vi "Test.vi"   [LabVIEW 2019]
doc: "This VI is called when test mode begins, and will automatically be terminated when it ends. You can add manual or automatic tests and invoke them from the dashboard."
uses:
  <vilib>/Rock Robotics/WPI/ThirdParty/Phoenix-LabVIEW/Motor Controller/Get/CTRE_Phoenix_MotorController_GetQuadratureData.vi
  <vilib>/Rock Robotics/WPI/Solenoid/Deprecated/WPI_SolenoidGetBool.vi
  <vilib>/Rock Robotics/WPI/Solenoid/WPI_SolenoidGetEnum.vi
types:
  T1 = typedef "WPI_SolenoidDevRef.ctl" = cluster{"DevStatus":errorcluster, "Pneumatics Control Module":u8, "Forward Solenoid Channel":T2, "Reverse Solenoid Channel":T2}
  T2 = typedef "WPI_SolenoidChannel.ctl" = enum8{"Solenoid 0", "Solenoid 1", "Solenoid 2", "Solenoid 3", "Solenoid 4", "Solenoid 5", "Solenoid 6", "Solenoid 7", "Invalid"}
  T3 = typedef "WPI_MotorControlDeviceRef.ctl" = cluster{"DeviceStatus":errorcluster, "Type":T4, "PWM":cluster{"PWM Channel":T5, "DeadBand":T6}, "CAN":cluster{"Device Number":u8, "SetOutput VI Ref":variant, "GetOutput VI Ref":variant, "Enable VI Ref":variant, "Disable VI Ref":variant, "Data":variant}, "Invert":bool, "DIO PWM":cluster{"PWM \"Enable\" Channel":T5, "DIOChannel":T7, "PWM Rate":dbl}}
  T4 = typedef "WPI_MotorControlType.ctl" = enum16{"PWM", "CAN", "DIO PWM"}
  T5 = typedef "FPGA_DIOPWMChannel.ctl" = enum8{"PWM 0", "PWM 1", "PWM 2", "PWM 3", "PWM 4", "PWM 5", "PWM 6", "PWM 7", "PWM 8", "PWM 9", "PWM MXP 0", "PWM MXP 1", "PWM MXP 2", "PWM MXP 3", "PWM MXP 4", "PWM MXP 5", "PWM MXP 6", "PWM MXP 7", "PWM MXP 8", "PWM MXP 9", "Invalid"}
  T6 = typedef "WPI_PWMDeadband.ctl" = cluster{"Name":string, "maxPositivePwm":i32, "minPositivePwm":i32, "centerPwm":i32, "maxNegativePwm":i32, "minNegativePwm":i32, "angularRange":u16}
  T7 = typedef "FPGA_DIOChannel.ctl" = enum8{"DIO 0", "DIO 1", "DIO 2", "DIO 3", "DIO 4", "DIO 5", "DIO 6", "DIO 7", "DIO 8", "DIO 9", "DIO MXP 0", "DIO MXP 1", "DIO MXP 2", "DIO MXP 3", "DIO MXP 4", "DIO MXP 5", "DIO MXP 6", "DIO MXP 7", "DIO MXP 8", "DIO MXP 9", "DIO MXP 10", "DIO MXP 11", "DIO MXP 12", "DIO MXP 13", "DIO MXP 14", "DIO MXP 15", "SPI Port CS1", "SPI Port CS2", "SPI Port CS3", "SPI Port MISO", "SPI Port MOSI", "Invalid"}
  T8 = typedef "WPI_SwitchDevRef.ctl" = cluster{"DevStatus":errorcluster, "DIO Channel":T7, "CntIndex":T9, "Normally Closed":bool}
  T9 = typedef "FPGA_CounterCtrSystemIndex.ctl" = enum8{"Ctr 0", "Ctr 1", "Ctr 2", "Ctr 3", "Ctr 4", "Ctr 5", "Ctr 6", "Ctr 7", "Invalid"}
  T10 = typedef "WPI_SolenoidValue.ctl" = enum16{"Off", "On", "Forward", "Reverse"}
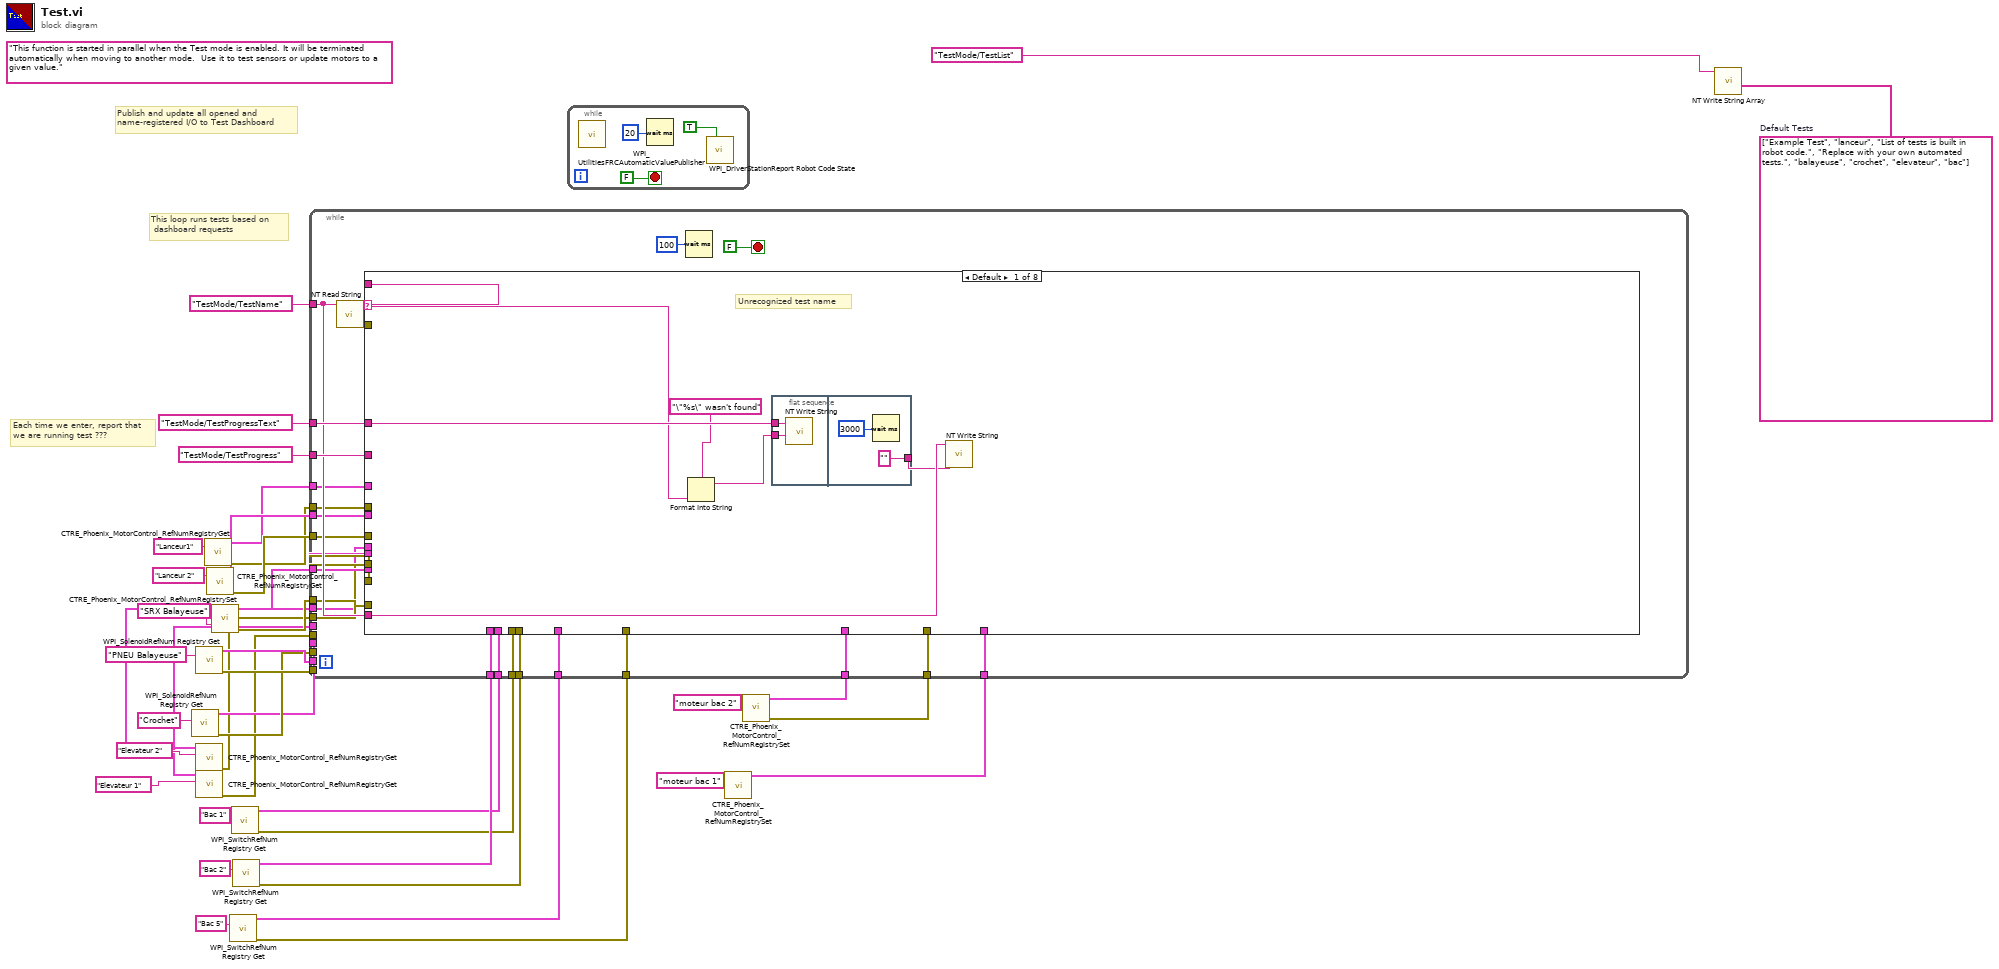
[diagram p0: block diagram]
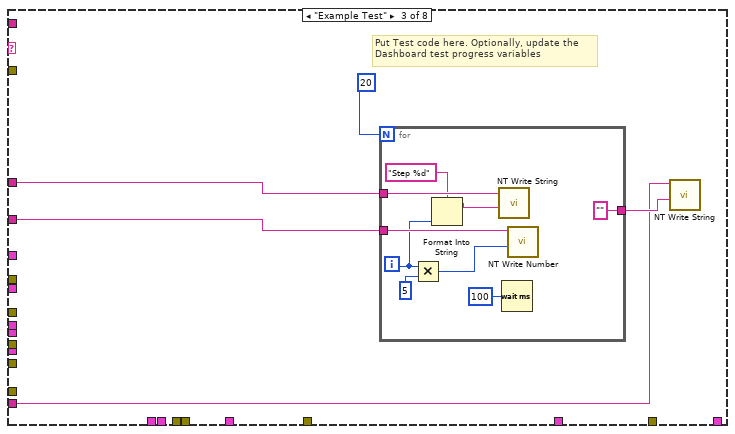
[diagram p3: hidden frame]
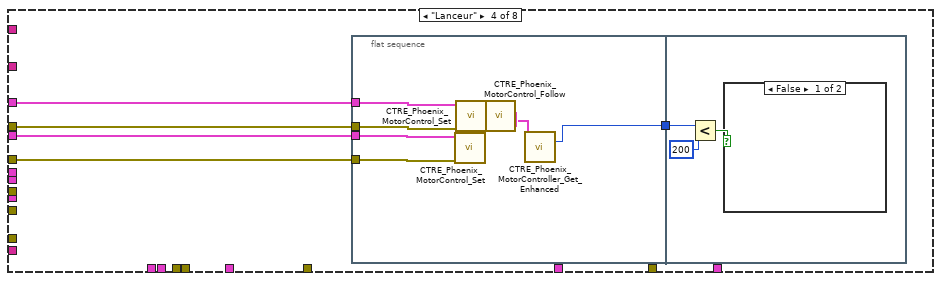
[diagram p4: hidden frame]
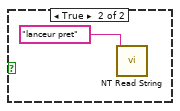
[diagram p5: hidden frame]
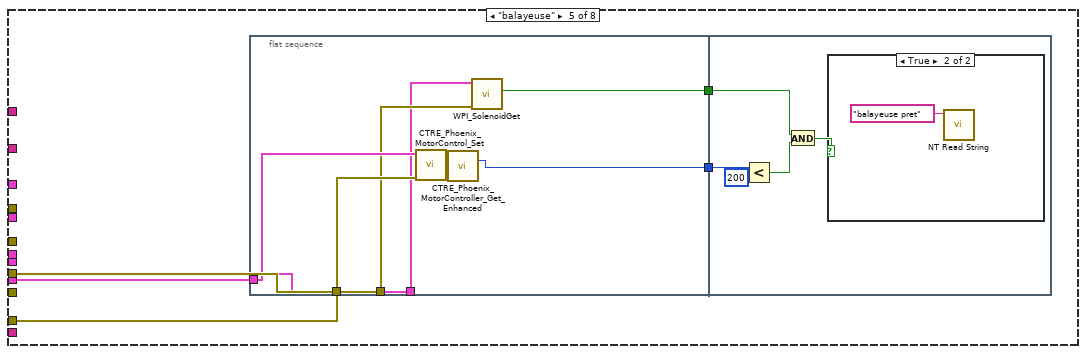
[diagram p6: hidden frame]
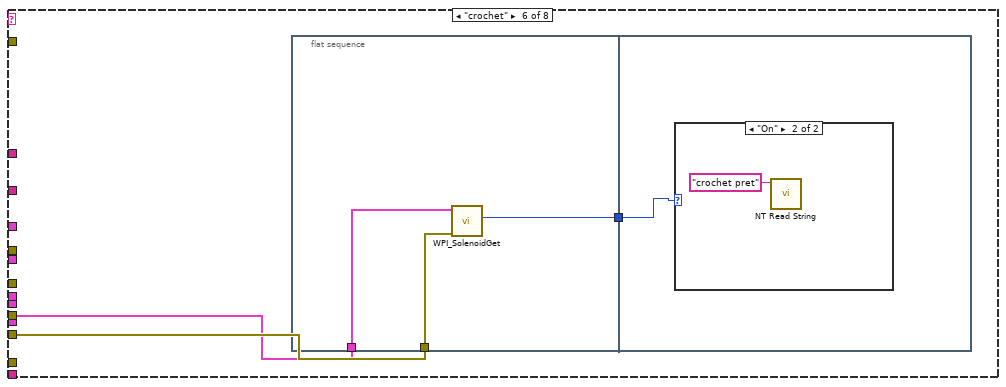
[diagram p8: hidden frame]
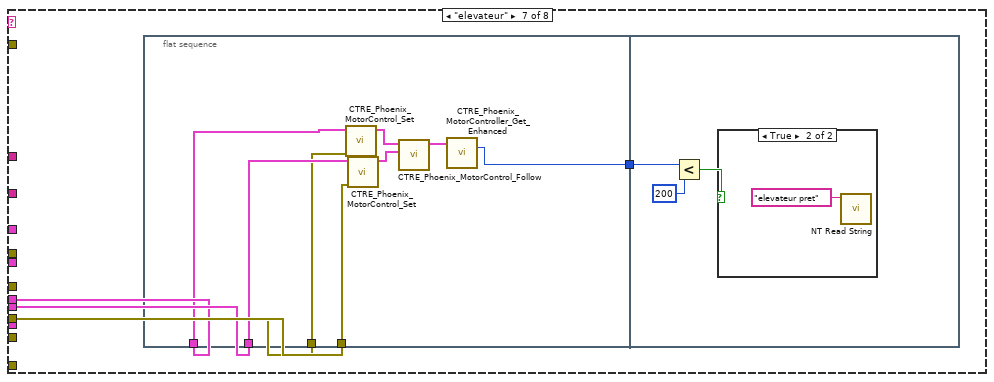
[diagram p10: hidden frame]
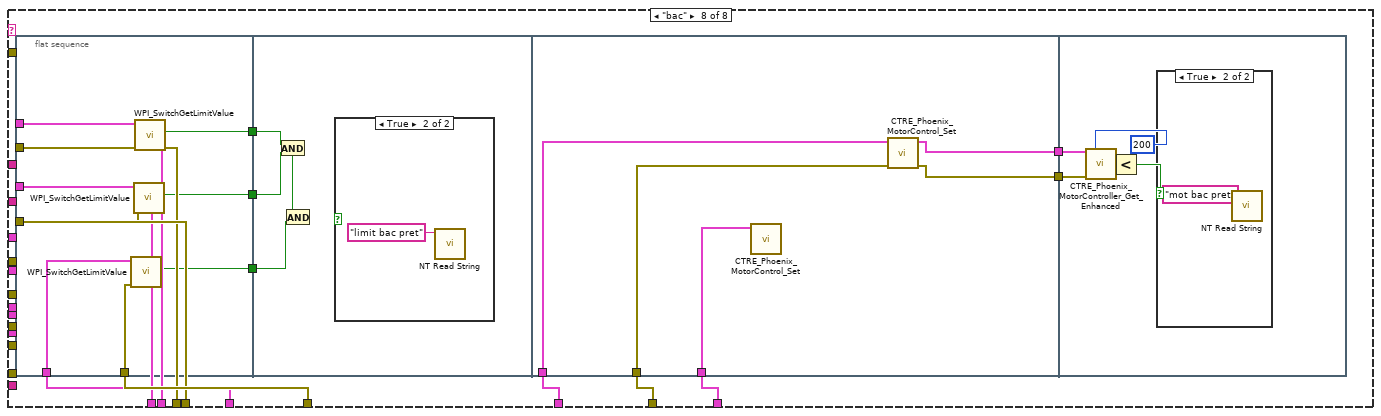
[diagram p12: hidden frame]
diagram:
  w37 = string[] ["Example Test", "lanceur", "List of tests is built in robot code.", "Replace with your own automated tests.", "balayeuse", "crochet", "elevateur", "bac"]  # Default Tests
  (unwired) "This function is started in parallel when the Test mode is enabled. It will be terminated automatically when moving to another mode.  Use it to test sensors or update motors to a given value."
  # "This loop runs tests based on \n dashboard requests"
  # "Publish and update all opened and\nname-registered I/O to Test Dashboard"
  # "Each time we enter, report that\nwe are running test ???"
  n1 = call <vilib>:"WPI_SolenoidRefNum Registry Get.vi"("refnum name"="Crochet") -> ("error out"=w22:errorcluster, "SolenoidDevRef"=w21:T1)  [unwired: 9 in]
  n2 = call <vilib>:"WPI_SolenoidRefNum Registry Get.vi"("refnum name"="PNEU Balayeuse") -> ("error out"=w25:errorcluster, "SolenoidDevRef"=w24:T1)  [unwired: 9 in]
  n3 = call <vilib>:"CTRE_Phoenix_MotorControl_RefNumRegistryGet.vi"("refnum name"="Elevateur 2") -> ("error out"=w16:errorcluster, "PhoenixMotorControlDevRef"=w15:T3)  [unwired: 9 in]
  n4 = call <vilib>:"CTRE_Phoenix_MotorControl_RefNumRegistryGet.vi"("refnum name"="Elevateur 1") -> ("error out"=w18:errorcluster, "PhoenixMotorControlDevRef"=w17:T3)  [unwired: 9 in]
  n5 = call <vilib>:"CTRE_Phoenix_MotorControl_RefNumRegistryGet.vi"("refnum name"="Lanceur1") -> ("error out"=w31:errorcluster, "PhoenixMotorControlDevRef"=w30:T3)  [unwired: 9 in]
  n6 = call <vilib>:"CTRE_Phoenix_MotorControl_RefNumRegistryGet.vi"("refnum name"="Lanceur 2") -> ("error out"=w33:errorcluster, "PhoenixMotorControlDevRef"=w32:T3)  [unwired: 9 in]
  n7 = call <vilib>:"CTRE_Phoenix_MotorControl_RefNumRegistrySet.vi"("refnum name"="SRX Balayeuse") -> ("error out"=w28:errorcluster, "PhoenixMotorControlDevRef"=w27:T3)  [unwired: 9 in]
  n8 = call <vilib>:"WPI_SwitchRefNum Registry Get.vi"("refnum name"="Bac 5") -> ("error out"=w11:errorcluster, "SwitchDevRef"=w10:T8)  [unwired: 9 in]
  n9 = call <vilib>:"WPI_SwitchRefNum Registry Get.vi"("refnum name"="Bac 1") -> ("error out"=w7:errorcluster, "SwitchDevRef"=w6:T8)  [unwired: 9 in]
  n10 = call <vilib>:"WPI_SwitchRefNum Registry Get.vi"("refnum name"="Bac 2") -> ("error out"=w9:errorcluster, "SwitchDevRef"=w8:T8)  [unwired: 9 in]
  n11 = while {
    stop <- FALSE stop-if-true
    n12 = call <vilib>:"WPI_UtilitiesFRCAutomaticValuePublisher.vi"() -> ()  [unwired: 12 in]
    n13 = Wait (ms)(milliseconds to wait=u32 20) -> ()  [unwired: 1 out]
    n14 = call <vilib>:"WPI_DriverStationReport Robot Code State.vi"("Test"=TRUE ("Autonomous")) -> ()  [unwired: 10 in, 1 out]
  }
  n15 = call <vilib>:"CTRE_Phoenix_MotorControl_RefNumRegistrySet.vi"("refnum name"="moteur bac 1") -> ("PhoenixMotorControlDevRef"=w3:T3)  [unwired: 9 in, 1 out]
  n16 = call <vilib>:"CTRE_Phoenix_MotorControl_RefNumRegistrySet.vi"("refnum name"="moteur bac 2") -> ("error out"=w2:errorcluster, "PhoenixMotorControlDevRef"=w1:T3)  [unwired: 9 in]
  n17 = while {
    tunnel: "TestMode/TestName" ("Name") -> [w68]
    tunnel: "TestMode/TestProgressText" ("Name") -> [w71]
    tunnel: "TestMode/TestProgress" ("Name") -> [w70]
    tunnel: w33 -> [w66]
    tunnel: w32 -> [w65]
    tunnel: w31 -> [w64]
    tunnel: w30 -> [w63]
    tunnel: w28 -> [w62]
    tunnel: w27 -> [w61]
    tunnel: w25 -> [w60]
    tunnel: w24 -> [w59]
    tunnel: w22 -> [w58]
    tunnel: w21 -> [w57]
    tunnel: w18 -> [w56]
    tunnel: w17 -> [w55]
    tunnel: w16 -> [w54]
    tunnel: w15 -> [w53]
    tunnel: w11 -> [w52]
    tunnel: w10 -> [w51]
    tunnel: w9 -> [w50]
    tunnel: w8 -> [w49]
    tunnel: w7 -> [w48]
    tunnel: w6 -> [w47]
    tunnel: w3 -> [w46]
    tunnel: w2 -> [w45]
    tunnel: w1 -> [w44]
    stop <- FALSE stop-if-true
    n18 = call <vilib>:"NT Read String.vi"("Name"=w68) -> ("error out"=w67:errorcluster, "String"=w69:string)  [unwired: 9 in]
    n19 = case shown="Default" w69 {
      selector: w69 -> [w78 _ _ _ _ _ _ _]
      tunnel: w68 -> [w75 _ w84 _ _ _ _ _]
      tunnel: w71 -> [w79 _ w87 _ _ _ _ _]
      tunnel: w70 -> [_ _ w88 _ _ _ _ _]
      tunnel: w69 -> [_ _ _ _ _ _ _ _]
      tunnel: w67 -> [_ _ _ _ _ _ _ _]
      tunnel: w66 -> [_ _ _ w102 _ _ _ _]
      tunnel: w65 -> [_ _ _ w101 _ _ _ _]
      tunnel: w64 -> [_ _ _ w100 _ _ _ _]
      tunnel: w63 -> [_ _ _ w99 _ _ _ _]
      tunnel: w62 -> [_ _ _ _ w120 _ _ _]
      tunnel: w61 -> [_ _ _ _ w119 _ _ _]
      tunnel: w60 -> [_ _ _ _ w118 _ _ _]
      tunnel: w59 -> [_ _ _ _ w117 _ _ _]
      tunnel: w58 -> [_ _ _ _ _ w136 _ _]
      tunnel: w57 -> [_ _ _ _ _ w135 _ _]
      tunnel: w56 -> [_ _ _ _ _ _ w146 _]
      tunnel: w55 -> [_ _ _ _ _ _ w145 _]
      tunnel: w54 -> [_ _ _ _ _ _ w144 _]
      tunnel: w53 -> [_ _ _ _ _ _ w143 _]
      tunnel: w52 -> [_ _ _ _ _ _ _ w172]
      tunnel: w51 -> [_ _ _ _ _ _ _ w171]
      tunnel: w50 -> [_ _ _ _ _ _ _ w170]
      tunnel: w49 -> [_ _ _ _ _ _ _ w169]
      tunnel: w48 -> [_ _ _ _ _ _ _ w168]
      tunnel: w47 -> [_ _ _ _ _ _ _ w167]
      tunnel: w46 -> [_ _ _ _ _ _ _ w163]
      tunnel: w45 -> [_ _ _ _ _ _ _ w162]
      tunnel: w44 -> [_ _ _ _ _ _ _ w161]
      frame Default {
        # "Unrecognized test name"
        n20 = Format Into String(format string="\"%s\" wasn't found" ("Name"), w78) -> (resulting string=w77:string)  [unwired: 2 in, 1 out]
        n21 = flat-sequence {
          tunnel: w79 -> [w80]
          tunnel: w77 -> [w81]
          tunnel: ["" ("Name")] -> w74
          frame #0 {
            n22 = call <vilib>:"NT Write String.vi"("String"=w81, "Name"=w80) -> ()  [unwired: 9 in, 1 out]
          }
          frame #1 {
            n23 = Wait (ms)(milliseconds to wait=u32 3000) -> ()  [unwired: 1 out]
          }
        }
        n24 = call <vilib>:"NT Write String.vi"("String"=w74, "Name"=w75) -> ()  [unwired: 9 in, 1 out]
      }
      frame "" {
        # "No test to run"
      }
      frame "Example Test" {
        # "Put Test code here. Optionally, update the\nDashboard test progress variables"
        n25 = for {
          N: 20 -> [_]
          tunnel: w88 -> [w97]
          tunnel: w87 -> [w95]
          tunnel: ["" ("String")] -> w85
          i -> [w92]
          n26 = Multiply(x=w92, y=u32 5 ("milliseconds to wait")) -> (x*y=w93:u32)
          n27 = Format Into String(format string="Step %d", w92) -> (resulting string=w90:string)  [unwired: 2 in, 1 out]
          n28 = call <vilib>:"NT Write String.vi"("String"=w90, "Name"=w95) -> ()  [unwired: 9 in, 1 out]
          n29 = Wait (ms)(milliseconds to wait=u32 100) -> ()  [unwired: 1 out]
          n30 = call <vilib>:"NT Write Number.vi"("Numeric"=w93, "Name"=w97) -> ()  [unwired: 9 in, 1 out]
        }
        n31 = call <vilib>:"NT Write String.vi"("String"=w85, "Name"=w84) -> ()  [unwired: 9 in, 1 out]
      }
      frame "Lanceur" {
        n32 = flat-sequence {
          tunnel: w102 -> [w107]
          tunnel: w101 -> [w106]
          tunnel: w100 -> [w105]
          tunnel: w99 -> [w104]
          tunnel: [w103] -> w98
          tunnel: w98 -> [w112]
          frame #0 {
            n33 = call <vilib>:"CTRE_Phoenix_MotorControl_Set.vi"("error in (no error)"=w107, "PhoenixMotorControlDevRef"=w106) -> ("PhoenixMotorControlDevRef"=w109:T3)  [unwired: 8 in, 1 out]
            n34 = call <vilib>:"CTRE_Phoenix_MotorControl_Set.vi"("error in (no error)"=w105, "PhoenixMotorControlDevRef"=w104) -> ("PhoenixMotorControlDevRef"=w110:T3)  [unwired: 8 in, 1 out]
            n35 = call <vilib>:"CTRE_Phoenix_MotorControl_Follow.vi"("Master Controller to Follow"=w109, "PhoenixMotorControlDevRef"=w110) -> ("PhoenixMotorControlDevRef"=w108:T3)  [unwired: 8 in, 1 out]
            n36 = call-poly <vilib>:"CTRE_Phoenix_MotorController_Get_Enhanced.vi"("PhoenixMotorControlDevRef"=w108) -> ("Quadrature Position"=w103:i32)  [unwired: 11 in, 3 out]
          }
          frame #1 {
            n37 = Less?(x=w112, y=200) -> (x < y?=w111:bool)
            n38 = case shown="False" w111 {
              frame False {
              }
              frame True {
                n39 = call <vilib>:"NT Read String.vi"("Name"="lanceur pret") -> ()  [unwired: 9 in, 2 out]
              }
            }
          }
        }
      }
      frame "balayeuse" {
        n40 = flat-sequence {
          tunnel: w120 -> [w126]
          tunnel: w119 -> [w125]
          tunnel: w118 -> [w124]
          tunnel: w117 -> [w123]
          tunnel: [w122] -> w116
          tunnel: [w121] -> w115
          tunnel: w116 -> [w131]
          tunnel: w115 -> [w129]
          frame #0 {
            n41 = call <vilib>:"CTRE_Phoenix_MotorControl_Set.vi"("error in (no error)"=w126, "PhoenixMotorControlDevRef"=w125) -> ("PhoenixMotorControlDevRef"=w127:T3)  [unwired: 8 in, 1 out]
            n42 = call-poly <vilib>:"CTRE_Phoenix_MotorController_Get_Enhanced.vi"("PhoenixMotorControlDevRef"=w127) -> ("Quadrature Position"=w122:i32)  [unwired: 11 in, 3 out]
            n43 = call-poly <vilib>:"WPI_SolenoidGet.vi"("error in (no error)"=w124, "SolenoidDevRef"=w123) -> ("Value"=w121:bool)  [unwired: 7 in, 2 out]
          }
          frame #1 {
            n44 = Less?(x=w131, y=200) -> (x < y?=w130:bool)
            n45 = And(x=w129, y=w130) -> (x .and. y?=w128:bool)
            n46 = case shown="True" w128 {
              frame False {
              }
              frame True {
                n47 = call <vilib>:"NT Read String.vi"("Name"="balayeuse pret") -> ()  [unwired: 9 in, 2 out]
              }
            }
          }
        }
      }
      frame "crochet" {
        n48 = flat-sequence {
          tunnel: w136 -> [w139]
          tunnel: w135 -> [w138]
          tunnel: [w137] -> w134
          tunnel: w134 -> [w140]
          frame #0 {
            n49 = call-poly <vilib>:"WPI_SolenoidGet.vi"("error in (no error)"=w139, "SolenoidDevRef"=w138) -> ("Value"=w137:T10)  [unwired: 7 in, 2 out]
          }
          frame #1 {
            n50 = case shown="\"On\"" w140 {
              frame "Off", Default {
              }
              frame "On" {
                n51 = call <vilib>:"NT Read String.vi"("Name"="crochet pret") -> ()  [unwired: 9 in, 2 out]
              }
            }
          }
        }
      }
      frame "elevateur" {
        n52 = flat-sequence {
          tunnel: w146 -> [w151]
          tunnel: w145 -> [w150]
          tunnel: w144 -> [w149]
          tunnel: w143 -> [w148]
          tunnel: [w147] -> w142
          tunnel: w142 -> [w156]
          frame #0 {
            n53 = call <vilib>:"CTRE_Phoenix_MotorControl_Set.vi"("error in (no error)"=w149, "PhoenixMotorControlDevRef"=w148) -> ("PhoenixMotorControlDevRef"=w154:T3)  [unwired: 8 in, 1 out]
            n54 = call <vilib>:"CTRE_Phoenix_MotorControl_Set.vi"("error in (no error)"=w151, "PhoenixMotorControlDevRef"=w150) -> ("PhoenixMotorControlDevRef"=w153:T3)  [unwired: 8 in, 1 out]
            n55 = call <vilib>:"CTRE_Phoenix_MotorControl_Follow.vi"("Master Controller to Follow"=w153, "PhoenixMotorControlDevRef"=w154) -> ("PhoenixMotorControlDevRef"=w152:T3)  [unwired: 8 in, 1 out]
            n56 = call-poly <vilib>:"CTRE_Phoenix_MotorController_Get_Enhanced.vi"("PhoenixMotorControlDevRef"=w152) -> ("Quadrature Position"=w147:i32)  [unwired: 11 in, 3 out]
          }
          frame #1 {
            n57 = Less?(x=w156, y=200) -> (x < y?=w155:bool)
            n58 = case shown="True" w155 {
              frame False {
              }
              frame True {
                n59 = call <vilib>:"NT Read String.vi"("Name"="elevateur pret") -> ()  [unwired: 9 in, 2 out]
              }
            }
          }
        }
      }
      frame "bac" {
        n60 = flat-sequence {
          tunnel: w172 -> [w181]
          tunnel: w171 -> [w180]
          tunnel: w170 -> [w179]
          tunnel: w169 -> [w178]
          tunnel: w168 -> [w177]
          tunnel: w167 -> [w176]
          tunnel: [w175] -> w166
          tunnel: [w174] -> w165
          tunnel: [w173] -> w164
          tunnel: w166 -> [w185]
          tunnel: w165 -> [w184]
          tunnel: w164 -> [w182]
          tunnel: w163 -> [w191]
          tunnel: w162 -> [w190]
          tunnel: w161 -> [w189]
          tunnel: [w188] -> w160
          tunnel: [w187] -> w159
          tunnel: w160 -> [w194]
          tunnel: w159 -> [w193]
          frame #0 {
            n61 = call <vilib>:"WPI_SwitchGetLimitValue.vi"("error in (no error)"=w181, "SwitchDevRef"=w180) -> ("Switch Pressed"=w173:bool)  [unwired: 7 in, 2 out]
            n62 = call <vilib>:"WPI_SwitchGetLimitValue.vi"("error in (no error)"=w179, "SwitchDevRef"=w178) -> ("Switch Pressed"=w174:bool)  [unwired: 7 in, 2 out]
            n63 = call <vilib>:"WPI_SwitchGetLimitValue.vi"("error in (no error)"=w177, "SwitchDevRef"=w176) -> ("Switch Pressed"=w175:bool)  [unwired: 7 in, 2 out]
          }
          frame #1 {
            n64 = And(x=w185, y=w184) -> (x .and. y?=w183:bool)
            n65 = And(x=w183, y=w182) -> ()  [unwired: 1 out]
            n66 = case shown="True" {
              selector: _ -> [_ _]
              frame False {
              }
              frame True {
                n67 = call <vilib>:"NT Read String.vi"("Name"="limit bac pret") -> ()  [unwired: 9 in, 2 out]
              }
            }
          }
          frame #2 {
            n68 = call <vilib>:"CTRE_Phoenix_MotorControl_Set.vi"("PhoenixMotorControlDevRef"=w191) -> ()  [unwired: 9 in, 2 out]
            n69 = call <vilib>:"CTRE_Phoenix_MotorControl_Set.vi"("error in (no error)"=w190, "PhoenixMotorControlDevRef"=w189) -> ("error out"=w187:errorcluster, "PhoenixMotorControlDevRef"=w188:T3)  [unwired: 8 in]
          }
          frame #3 {
            n70 = call-poly <vilib>:"CTRE_Phoenix_MotorController_Get_Enhanced.vi"("PhoenixMotorControlDevRef"=w194, "error in"=w193) -> ("Quadrature Position"=w196:i32)  [unwired: 10 in, 3 out]
            n71 = Less?(x=w196, y=200) -> (x < y?=w192:bool)
            n72 = case shown="True" w192 {
              frame False {
              }
              frame True {
                n73 = call <vilib>:"NT Read String.vi"("Name"="mot bac pret") -> ()  [unwired: 9 in, 2 out]
              }
            }
          }
        }
      }
    }
    n74 = Wait (ms)(milliseconds to wait=u32 100) -> ()  [unwired: 1 out]
  }
  n75 = call <vilib>:"NT Write String Array.vi"("String Array"=w37, "Name"="TestMode/TestList") -> ()  [unwired: 9 in, 1 out]
